vi "FlatToRichni_measurementlink_pinmap_v1_QueryRelaysResponse.vi"(5 "OutputClusterType":T1, 11 "InputCluster":T4) -> (3 "OutputCluster":T1)   [LabVIEW 2020, in "ni.measurementlink.pinmap.v1.api.lvlib"]
uses:
  ni.measurementlink.pinmap.v1.api.lvlib
  ni_measurementlink_pinmap_v1_QueryRelaysResponse_Flat.ctl
  ni_measurementlink_pinmap_v1_RelayDefinition_Flat.ctl
  ni_measurementlink_pinmap_v1_RelayGroupDefinition_Flat.ctl
  ni_measurementlink_pinmap_v1_QueryRelaysResponse.ctl
  ni_measurementlink_pinmap_v1_RelayDefinition.ctl
  ni_measurementlink_pinmap_v1_RelayGroupDefinition.ctl
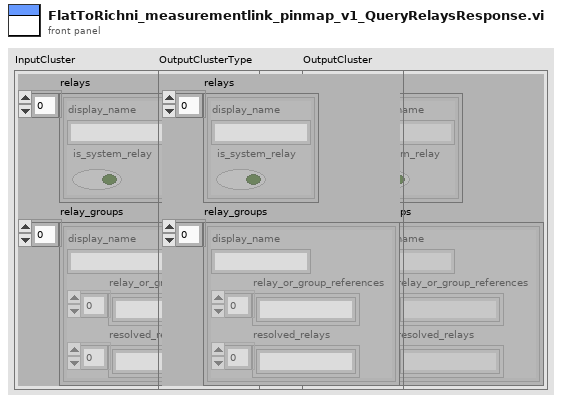
[diagram p1: front panel]
types:
  T1 = typedef "ni.measurementlink.pinmap.v1.api.lvlib/ni_measurementlink_pinmap_v1_QueryRelaysResponse.ctl" = cluster{"relays":T2[], "relay_groups":T3[]}
  T2 = typedef "ni.measurementlink.pinmap.v1.api.lvlib/ni_measurementlink_pinmap_v1_RelayDefinition.ctl" = cluster{"display_name":string, "is_system_relay":bool}
  T3 = typedef "ni.measurementlink.pinmap.v1.api.lvlib/ni_measurementlink_pinmap_v1_RelayGroupDefinition.ctl" = cluster{"display_name":string, "relay_or_group_references":string[], "resolved_relays":string[]}
  T4 = typedef "ni.measurementlink.pinmap.v1.api.lvlib/ni_measurementlink_pinmap_v1_QueryRelaysResponse_Flat.ctl" = cluster{"relays":T5[], "relay_groups":T6[]}
  T5 = typedef "ni.measurementlink.pinmap.v1.api.lvlib/ni_measurementlink_pinmap_v1_RelayDefinition_Flat.ctl" = cluster{"display_name":string, "is_system_relay":bool}
  T6 = typedef "ni.measurementlink.pinmap.v1.api.lvlib/ni_measurementlink_pinmap_v1_RelayGroupDefinition_Flat.ctl" = cluster{"display_name":string, "relay_or_group_references":string[], "resolved_relays":string[]}
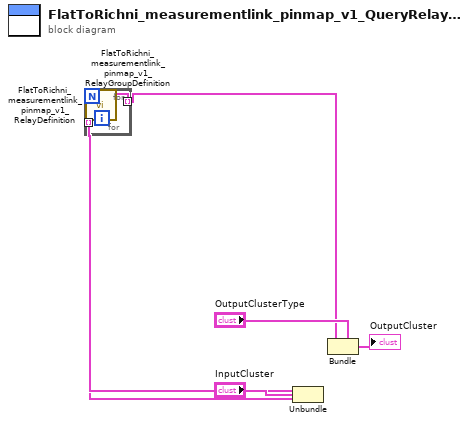
[diagram p0: block diagram]
diagram:
  n1 = Unbundle "Unbundle"("InputCluster") -> ("relays"=w4:T5[], "relay_groups"=w2:T6[])
  n2 = for {
    tunnel: w2 -> [w9] mode=indexing
    tunnel: [w8] -> w1 mode=indexing
    n3 = call "FlatToRichni_measurementlink_pinmap_v1_RelayGroupDefinition.vi"("InputCluster"=w9) -> ("OutputCluster"=w8:T3)  [unwired: 10 in]
  }
  n4 = for {
    tunnel: w4 -> [w11] mode=indexing
    tunnel: [w10] -> w3 mode=indexing
    n5 = call "FlatToRichni_measurementlink_pinmap_v1_RelayDefinition.vi"("InputCluster"=w11) -> ("OutputCluster"=w10:T2)  [unwired: 10 in]
  }
  n6 = Bundle "Bundle"(cluster="OutputClusterType", "relays"=w3, "relay_groups"=w1) -> (→"OutputCluster":T1)
